vi "enviotiempo.vi"(8 "fin de cadena":string=" S", 11 "x":i32) -> (2 "String":string, 5 "ok":bool)   [LabVIEW 2017]
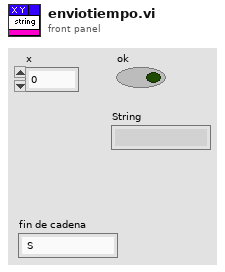
[diagram p1: front panel]
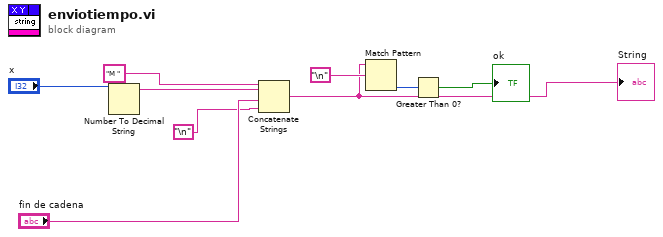
[diagram p0: block diagram]
diagram:
  n1 = Number To Decimal String(number="x") -> (decimal integer string=w5:string)  [unwired: 1 in]
  n2 = Concatenate Strings("M " ("string"), w5, "fin de cadena", "\n") -> (w6:string)
  "String" <- w6
  n3 = Match Pattern(string=w6, regular expression="\n") -> (offset past match=w8:i32)  [unwired: 1 in, 3 out]
  n4 = Greater Than 0?(x=w8) -> (x > 0?=→"ok":bool)
